vi "SetHistogramParameter.vi"(7 "tacq":i32, 8 "error in (no error)":errorcluster, 9 "Value":i32, 10 "Parameter":enum16{"HistoLen", "HistoOffset", "Binning"}(ring)=enum."Binning", 11 "Multiharp in":refnum<class "Multiharp.lvclass">) -> (0 "error out":errorcluster, 3 "Multiharp out":refnum<class "Multiharp.lvclass">)   [LabVIEW 2023, in "Multiharp.lvlib" / "Multiharp.lvclass"]
uses:
  Multiharp.lvclass
  Multiharp.lvclass/Multiharp.ctl
panel:
  in  "event data":cluster{"ActualHistoLe":i32}
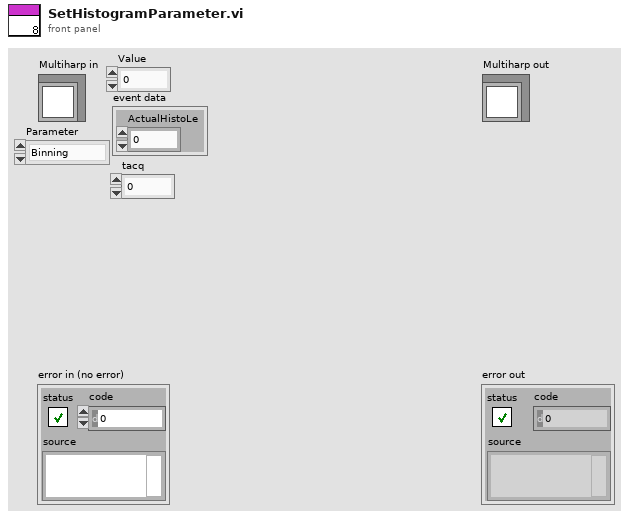
[diagram p1: front panel]
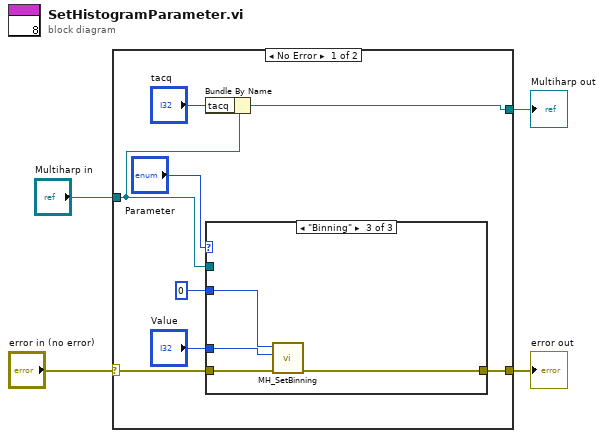
[diagram p0: block diagram]
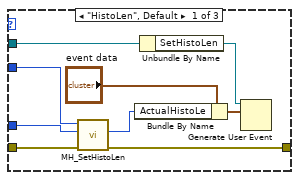
[diagram p2: hidden frame]
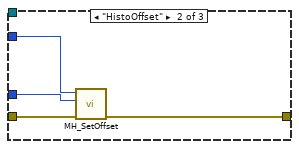
[diagram p3: hidden frame]
diagram:
  n1 = case shown="No Error" "error in (no error)" {
    selector: "error in (no error)" -> [w10 w31]
    tunnel: [w8 w31] -> w3
    tunnel: [w5 w30] -> w1
    tunnel: "Multiharp in" -> [w6 w30]
    frame No Error {
      n2 = Bundle By Name(cluster=w6, "tacq"="tacq") -> (w5:refnum<class "Multiharp.lvclass">)
      n3 = case shown="\"Binning\"" "Parameter" {
        tunnel: 0 ("devidx") -> [w18 w25 w29]
        tunnel: "Value" -> [w19 w24 w28]
        tunnel: w10 -> [w21 w23 w27]
        tunnel: [w20 w22 w26] -> w8
        tunnel: w6 -> [w16 _ _]
        frame "HistoLen", Default {
          n4 = call "MH_SetHistoLen.vi"("error in (no error)"=w21, "lencode"=w19, "devidx"=w18) -> ("error out"=w20:errorcluster, "actuallen"=w15:i32)  [unwired: 6 in, 1 out]
          n5 = Bundle By Name(cluster="event data", "ActualHistoLe"=w15) -> (w13:cluster{"ActualHistoLe":i32})
          n6 = Unbundle By Name(w16) -> ("SetHistoLen"=w17:refnum<user-event>)
          n7 = Generate User Event(user event=w17, event data cluster=w13) -> ()  [unwired: 2 in, 2 out]
        }
        frame "HistoOffset" {
          n8 = call "MH_SetOffset.vi"("error in (no error)"=w23, "Offset"=w24, "devidx"=w25) -> ("error out"=w22:errorcluster)  [unwired: 7 in, 1 out]
        }
        frame "Binning" {
          n9 = call "MH_SetBinning.vi"("error in (no error)"=w27, "Binning"=w28, "devidx"=w29) -> ("error out"=w26:errorcluster)  [unwired: 7 in, 1 out]
        }
      }
    }
    frame Error {
    }
  }
  "error out" <- w3
  "Multiharp out" <- w1
